vi "PID Online Autotuning (Step Closed Loop).vi"(0 "setpoint":dbl(slide)=30.8641975308642 scale=0.0..100.0 scale format="%.1f", 1 "manipulated variable":dbl(slide)=30.8641975308642 scale=0.0..100.0 scale format="%.1f", 3 "autotuning parameters":T2={"type of controller"=0, "relay cycles"=3, "relay amplitude"=1.0, "control specifications"=2, "PV noise level"=0.1} {"PV noise level" format="%.2f"; "control specifications" items=["normal", "fast", "slow"]; "relay amplitude" format="%.2f"; "type of controller" items=["P", "PI", "PID"]}, 5 "process variable":dbl(slide)=19.583333333333336 scale=0.0..100.0 scale format="%.1f", 9 "PID gains in":T1={"proportional gain (Kc)"=1.0, "integral time (Ti, min)"=0.01, "derivative time (Td, min)"=0.0} {"derivative time (Td, min)" format="%.3f"; "integral time (Ti, min)" format="%.3f"; "proportional gain (Kc)" format="%.3f"}, 11 "dt (s)":dbl=-1.0 format="%.3f", 12 "reinitialize? (F)":bool, 13 "autotune? (F)":bool) -> (4 "setpoint out":dbl(slide)=30.8641975308642 scale=0.0..100.0 scale format="%.1f", 6 "process variable out":dbl(slide)=19.583333333333336 scale=0.0..100.0 scale format="%.1f", 8 "tuning completed?":bool, 10 "PID gains out":T1={"proportional gain (Kc)"=1.0, "integral time (Ti, min)"=0.01, "derivative time (Td, min)"=0.0} {"derivative time (Td, min)" format="%.3f"; "integral time (Ti, min)" format="%.3f"; "proportional gain (Kc)" format="%.3f"}, 14 "tuned PID gains":T1={"proportional gain (Kc)"=1.0, "integral time (Ti, min)"=0.01, "derivative time (Td, min)"=0.0} {"derivative time (Td, min)" format="%.3f"; "integral time (Ti, min)" format="%.3f"; "proportional gain (Kc)" format="%.3f"})   [LabVIEW 2020, in "NI_PID_autopid.lvlib"]
doc: "Controls the parameters of a PID controller based on the autotuning technique of the polymorphic instance you select. You can use this VI in applications with other PID VIs, such as PID or PID Advanced, to construct and tune a PID controller. You must manually select the polymorphic instance to use."
uses:
  <vilib>/addons/control/pid/NI_PID_autopid.lvlib
  <vilib>/addons/control/pid/autopid.llb/PID autotuning parameters.ctl
  <vilib>/addons/control/pid/autopid.llb/PID Autotuning Design (Auto).vi
  <vilib>/addons/control/pid/NI_PID_pid.lvlib
  <vilib>/ptbypt/NI_PtbyPt.lvlib
panel:
  # "Closed Loop Step Response"
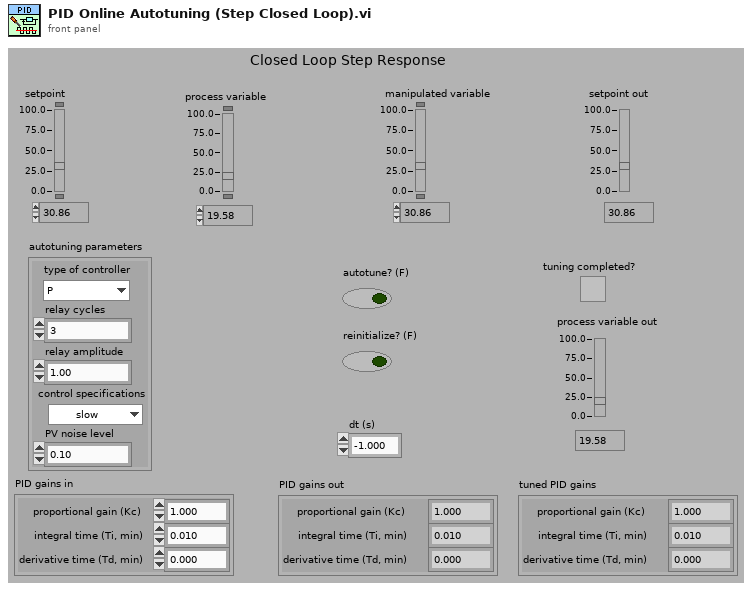
[diagram p1: front panel]
types:
  T1 = cluster{"proportional gain (Kc)":dbl, "integral time (Ti, min)":dbl, "derivative time (Td, min)":dbl}
  T2 = typedef "PID autotuning parameters.ctl" = cluster{"type of controller":u16, "relay cycles":i32, "relay amplitude":dbl, "control specifications":u16, "PV noise level":dbl}
  T3 = cluster{"Plant Gain (K)":dbl, "Time Constant (T)":dbl, "Dead Time (L)":dbl}
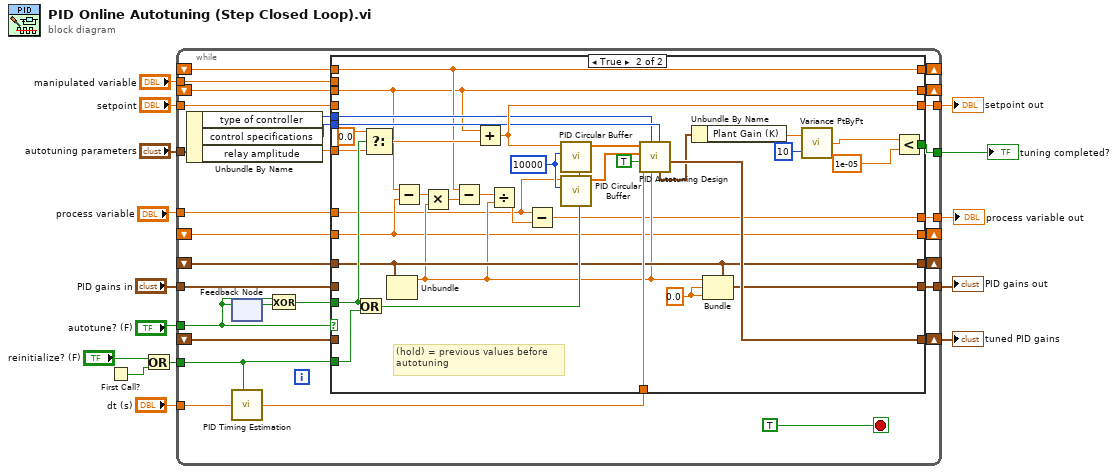
[diagram p0: block diagram]
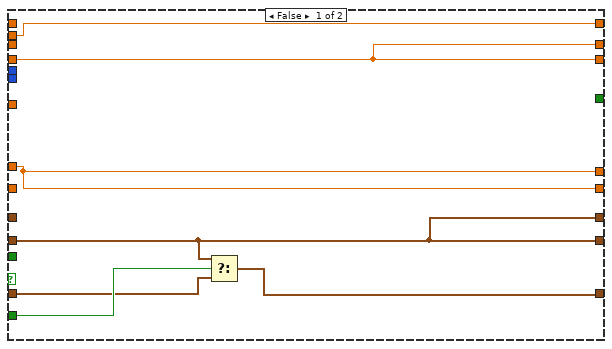
[diagram p2: hidden frame]
diagram:
  n1 = First Call?() -> (First Call?: T/F=w13:bool)
  n2 = Or(x="reinitialize? (F)", y=w13) -> (x .or. y?=w8:bool)
  n3 = while {
    tunnel: w8 -> [w37]
    tunnel: "dt (s)" -> [w43]
    tunnel: "process variable" -> [w38]
    tunnel: "autotuning parameters" -> [w41]
    tunnel: "PID gains in" -> [w32]
    tunnel: "setpoint" -> [w36]
    tunnel: "autotune? (F)" -> [w28]
    tunnel: "manipulated variable" -> [w40]
    tunnel: [w35] -> w5
    shift-right: [w34] -> _
    shift-left: _ -> [w33]
    tunnel: [w31] -> w4
    tunnel: [w30] -> w3
    shift-right: [w24] -> w2
    shift-left: _ -> [w23]
    shift-right: [w22] -> _
    shift-left: _ -> [w21]
    shift-right: [w20] -> _
    shift-left: _ -> [w19]
    shift-right: [w18] -> _
    shift-left: _ -> [w17]
    tunnel: [w16] -> w1
    stop <- TRUE stop-if-true
    n4 = Unbundle By Name(w41) -> ("type of controller"=w26:u16, "control specifications"=w25:u16, "relay amplitude"=w42:dbl)
    n5 = feedback #1() -> (w29:bool)  [unwired: 1 in]
    n6 = feedback-in #1(w28) -> ()
    n7 = call <vilib>:"PID Timing Estimation.vi"("Initialize?"=w37, "dt (s) in"=w43) -> ("dt (s) out"=w39:dbl)  [unwired: 7 in]
    n8 = Exclusive Or(1:w29, 2:w28) -> (0:w27:bool)
    n9 = case shown="True" w28 {
      tunnel: w42 -> [_ w72]
      tunnel: w40 -> [w45 _]
      tunnel: w39 -> [_ w76]
      tunnel: w38 -> [w47 w59]
      tunnel: w37 -> [w51 w82]
      tunnel: [w48 w79] -> w35
      tunnel: w36 -> [w48 _]
      tunnel: [w48 w58] -> w34
      tunnel: w33 -> [_ w58]
      tunnel: [w46 w69] -> w31
      tunnel: w32 -> [w46 _]
      tunnel: [w47 w60] -> w30
      tunnel: w27 -> [_ w80]
      tunnel: w26 -> [_ w74]
      tunnel: w25 -> [_ w75]
      tunnel: [w50 w73] -> w24
      tunnel: w23 -> [w49 _]
      tunnel: [w47 w61] -> w22
      tunnel: w21 -> [_ w61]
      tunnel: [w46 w68] -> w20
      tunnel: w19 -> [_ w68]
      tunnel: [w45 w64] -> w18
      tunnel: w17 -> [_ w64]
      tunnel: [_ w52] -> w16
      frame False {
        n10 = Select(t=w46, s=w51, f=w49) -> (s? t:f=w50:T1)
      }
      frame True {
        w71 = 0.0 ("derivative time (Td, min)")
        w83 = 10000 ("sample length")
        # "(hold) = previous values before \nautotuning"
        n11 = Or(x=w80, y=w82) -> (x .or. y?=w81:bool)
        n12 = Select(t=0.0, s=w80, f=w72) -> (s? t:f=w84:dbl)
        n13 = Unbundle(w68) -> ("proportional gain (Kc)"=w65:dbl)  [unwired: 2 out]
        n14 = Subtract(x=w58, y=w61) -> (x-y=w67:dbl)
        n15 = Multiply(x=w67, y=w65) -> (x*y=w66:dbl)
        n16 = Subtract(x=w64, y=w66) -> (x-y=w63:dbl)
        n17 = Add(x=w58, y=w84) -> (x+y=w79:dbl)
        n18 = Divide(x=w63, y=w65) -> (x/y=w62:dbl)
        n19 = Subtract(x=w59, y=w62) -> (x-y=w60:dbl)
        n20 = call <vilib>:"PID Circular Buffer.vi"("initialize"=w81, "sample length"=w83, "input data point"=w79) -> ("Current Queue"=w78:dbl[])  [unwired: 7 in, 1 out]
        n21 = call <vilib>:"PID Circular Buffer.vi"("initialize"=w81, "sample length"=w83, "input data point"=w59) -> ("Current Queue"=w77:dbl[])  [unwired: 7 in, 1 out]
        n22 = call-poly <vilib>:"PID Autotuning Design.vi"("Ziegler-Nichols Speed"=w75, "Controller Gain (K)"=w65, "Type of Controller"=w74, "dt (s)"=w76, "closed-loop?"=TRUE, "Response signal"=w77, "Stimulus signal"=w78) -> ("PID gains"=w73:T1, "Plant Parameters"=w53:T3)  [unwired: 1 in, 2 out]
        n23 = Unbundle By Name(w53) -> ("Plant Gain (K)"=w57:dbl)
        n24 = Bundle(cluster=w68, "proportional gain (Kc)"=w65, "integral time (Ti, min)"=w71, "derivative time (Td, min)"=w71) -> (w69:T1)
        n25 = call <vilib>:"Variance PtByPt.vi"("x"=w57, "sample length"=10) -> ("variance"=w55:dbl)  [unwired: 1 in, 2 out]
        n26 = Less?(x=w55, y=1e-05) -> (x < y?=w52:bool)
      }
    }
  }
  "PID gains out" <- w4
  "process variable out" <- w3
  "setpoint out" <- w5
  "tuning completed?" <- w1
  "tuned PID gains" <- w2
